vi "RegEx_Hdot.vi"(11 "Hdot String":string="0.50E-5 Sv/h 04 %  ") -> (2 "Error in %":dbl, 3 "Hdot dbl (uSv/s)":dbl)   [LabVIEW 2014]
uses:
  <vilib>/regexp/Match Regular Expression.xnode
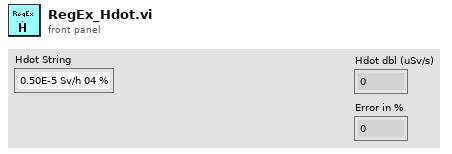
[diagram p1: front panel]
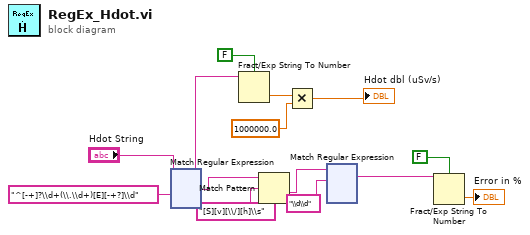
[diagram p0: block diagram]
diagram:
  n1 = xnode "Match Regular Expression"("input string"="Hdot String", "regular expression"="^[-+]?\\d+(\\.\\d+)[E][-+?]\\d") -> ("whole match"=w12:string, "after match"=w10:string)  [unwired: 4 in, 3 out]
  n2 = Fract/Exp String To Number(use system decimal point (T)=FALSE, string=w12) -> (number=w3:dbl)  [unwired: 2 in, 1 out]
  n3 = Match Pattern(string=w10, regular expression="[S][v][\\/][h]\\s") -> (after substring=w8:string)  [unwired: 1 in, 3 out]
  n4 = Multiply(x=w3, y=1000000.0) -> (x*y=→"Hdot dbl (uSv/s)":dbl)
  n5 = xnode "Match Regular Expression"("input string"=w8, "regular expression"="\\d\\d") -> ("whole match"=w4:string)  [unwired: 4 in, 4 out]
  n6 = Fract/Exp String To Number(use system decimal point (T)=FALSE, string=w4) -> (number=→"Error in %":dbl)  [unwired: 2 in, 1 out]
